vi "Receive Message.vi"(6 "priority":i32, 10 "RPI.SenseHat.Actor in":refnum<class "RPI.SenseHat.Actor.lvclass">, 11 "Message in":refnum<class "Message.lvclass">) -> (0 "error out":errorcluster, 2 "Actor out":refnum<class "Actor.lvclass">)   [LabVIEW 2020, in "RPI.SenseHat.Actor.lvlib" / "RPI.SenseHat.Actor.lvclass"]
doc: "This VI should be overriden ONLY if you are creating a proxy actor for remote transmission. If you are, override this VI to transmit the received message to a new destination, maintaining the given priority."
uses:
  <vilib>/ActorFramework/Message/Message.lvclass
  <vilib>/ActorFramework/Actor/Actor.lvclass
  RPI.SenseHat.Actor.lvclass
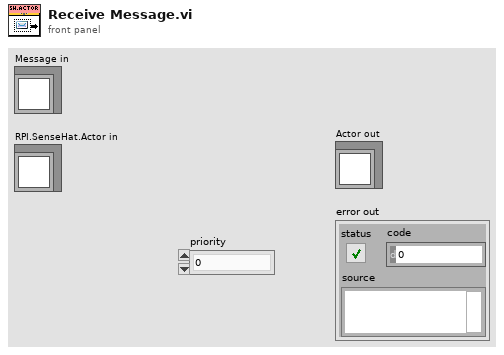
[diagram p1: front panel]
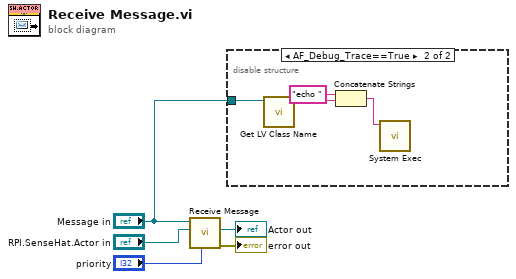
[diagram p0: block diagram]
diagram:
  n1 = call-parent "Receive Message.vi"("priority"="priority", "Actor in"="RPI.SenseHat.Actor in", "Message in"="Message in") -> ("error out"=→"error out":errorcluster, "Actor out"=→"Actor out":refnum<class "Actor.lvclass">)  [unwired: 7 in]
  n2 = disable-structure shown="AF_Debug_Trace==True" {
    disable-tunnel: "Message in" -> [_ w9]
    frame condition #0 {
    }
    frame condition #1 (active) {
      n3 = call <vilib>:"Get LV Class Name.vi"("object"=w9) -> ("class name"=w8:string)  [unwired: 9 in, 1 out]
      n4 = Concatenate Strings("echo " ("string"), w8) -> (w6:string)
      n5 = call <vilib>:"System Exec.vi"("command line"=w6) -> ()  [unwired: 7 in, 4 out]
    }
  }
